vi "PathPlanning.vi"(7 "Goal":cluster{"X":i16, "Y":i16}, 8 "error in":errorcluster, 9 "Corners":cluster{"Col":i16, "Row":i16}[](array[cluster]), 10 "Map":i8[][](array[numeric]), 11 "Robot in map":cluster{"Col":i16, "Row":i16}) -> (0 "error out":errorcluster, 2 "PathPoints":T1)   [LabVIEW 2009, in "Main.lvlib"]
doc: "Main path planning algorithm. Calculates path to the goal from map information."
uses:
  Main.lvlib
  Navigation/Nav_CordinateArray.ctl
  Navigation.lvlib
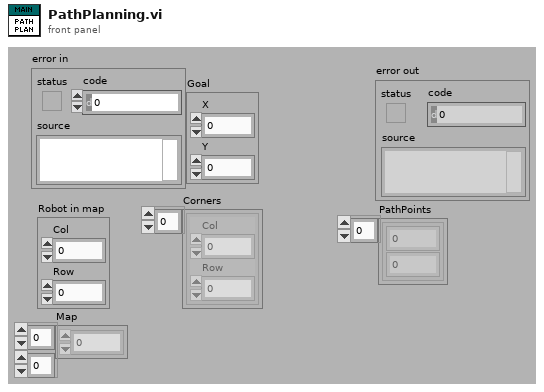
[diagram p1: front panel]
types:
  T1 = typedef "Navigation.lvlib/Nav_CordinateArray.ctl" = cluster{"X position":dbl, "Y position":dbl}[]
  T2 = cluster{"Robot":cluster{"X":i16, "Y":i16, "Bearing":dbl}, "Map":i8[][], "Goal":cluster{"X":i16, "Y":i16}, "Corners":cluster{"X":i16, "Y":i16}[]}
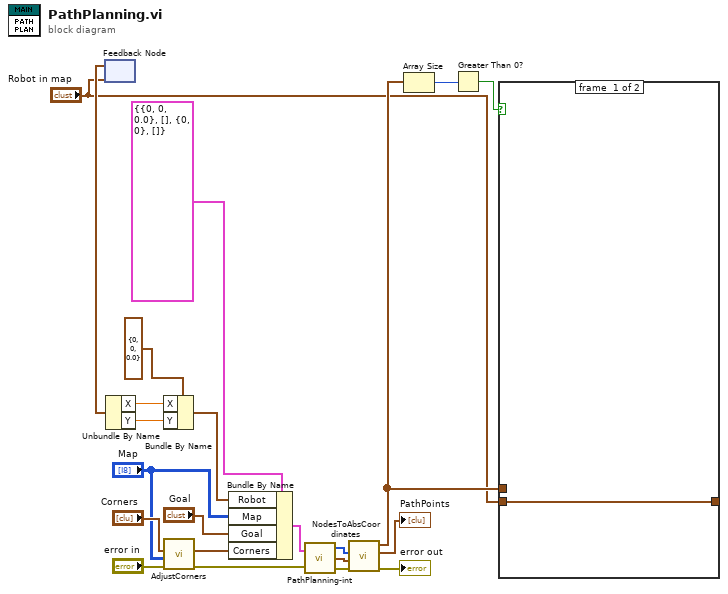
[diagram p0: block diagram]
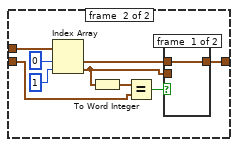
[diagram p2: hidden frame]
diagram:
  n1 = feedback #1("Robot in map") -> (w7:cluster{"X":dbl, "Y":dbl})
  n2 = Unbundle By Name(w7) -> ("X"=w2:dbl, "Y"=w1:dbl)
  n3 = Bundle By Name(cluster=cluster{"X":i16, "Y":i16, "Bearing":dbl} {"X"=0, "Y"=0, "Bearing"=0.0} ("Robot"), "X"=w2, "Y"=w1) -> (w8:cluster{"X":i16, "Y":i16, "Bearing":dbl})
  n4 = call "AdjustCorners.vi"("error in"="error in", "Map"="Map", "Corners"="Corners") -> ("error out"=w14:errorcluster, "Corners out"=w12:cluster{"Col":i16, "Row":i16}[])  [unwired: 7 in]
  n5 = Bundle By Name(cluster=T2 {"Robot"={"X"=0, "Y"=0, "Bearing"=0.0}, "Map"=[], "Goal"={"X"=0, "Y"=0}, "Corners"=[]} ("Map&Nodes"), "Robot"=w8, "Map"="Map", "Goal"="Goal", "Corners"=w12) -> (w17:T2)
  n6 = call "PathPlanning-int.vi"("Map&Nodes"=w17, "error in (no error)"=w14) -> ("Path"=w19:i32[], "Coordinates"=w20:cluster{"X":dbl, "Y":dbl}[], "error out"=w21:errorcluster)
  n7 = call "NodesToAbsCoordinates.vi"("error in"=w21, "Coordinates"=w20, "Path"=w19) -> ("error out"=→"error out":errorcluster, "Points output"=→"PathPoints":T1, "Map_Points"=w6:cluster{"X":dbl, "Y":dbl}[])  [unwired: 6 in]
  n8 = Array Size(array=w6) -> (size(s)=w5:i32)
  n9 = Greater Than 0?(x=w5) -> (x > 0?=w4:bool)
  n10 = case shown="True" w4 {
    tunnel: [w24 w33] -> w9
    tunnel: w6 -> [_ w30]
    tunnel: "Robot in map" -> [w24 w28]
    frame #0 {
    }
    frame #1 {
      n11 = Index Array(array=w30, index #1=0 ("index"), index #2=1 ("index")) -> (element #1=w29:cluster{"X":dbl, "Y":dbl}, element #2=w27:cluster{"X":dbl, "Y":dbl})
      n12 = To Word Integer(number=w27) -> (16bit integer=w26:cluster{"X":i16, "Y":i16})
      n13 = Equal?(x=w26, y=w28) -> (x = y?=w25:bool)
      n14 = case shown="True" w25 {
        tunnel: [w34 w35] -> w33
        tunnel: w29 -> [w34 _]
        tunnel: w27 -> [_ w35]
        frame #0 {
        }
        frame #1 {
        }
      }
    }
  }
